vi "LoadDBCFile.vi"(10 "Signals.In":T1(array[cluster]), 11 "DbcFilePath":path caption="選擇DBC檔案") -> (1 "Signal.Out":T1(array[cluster]), 2 "Path.out":path, 3 "OK?":bool)   [LabVIEW 2024]
uses:
  LoadDBCStep.ctl
panel:
  out "Exit":bool
  in  "Signals":T1(array[cluster])
  in  "Cancel Button":bool
  in  "OK Button":bool
  in  "RemoveItem":bool
  in  "AddItem":bool
  in  "SelectedSignalName":i32(listbox) caption="顯示資料欄位"
  in  "AllSignalName":i32(listbox) caption="所有資料欄位"
  in  "LoadSignal":bool
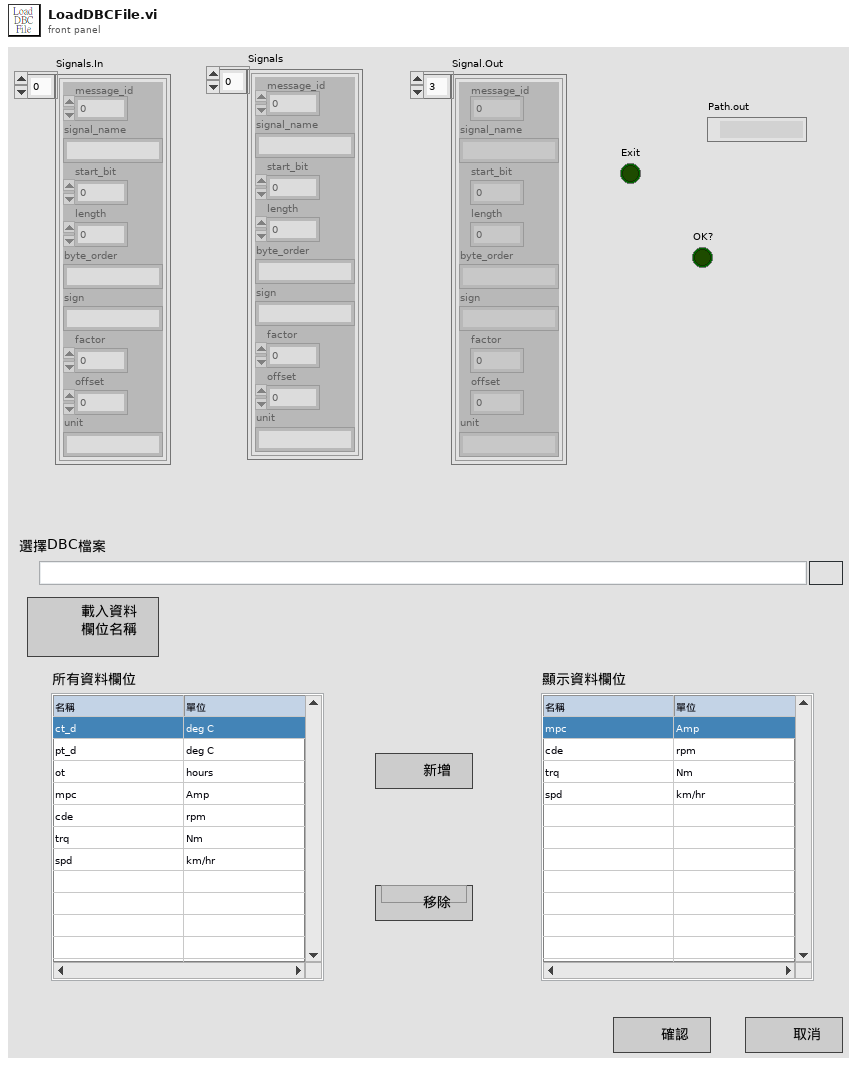
[diagram p1: front panel]
types:
  T1 = cluster{"message_id":i32, "signal_name":string, "start_bit":i32, "length":i32, "byte_order":string, "sign":string, "factor":dbl, "offset":dbl, "unit":string}[]
  T2 = typedef "LoadDBCStep.ctl" = enum16{"Idle", "Initialization", "OK Pressed", "Cancel Pressed", "LoadSignals", "AddItem", "RemoveItem", "UpdateSignalNameTable", "UpdateSelectedSignalNameTable", "End"}
  T3 = cluster{"message_id":i32, "signal_name":string, "start_bit":i32, "length":i32, "byte_order":string, "sign":string, "factor":dbl, "offset":dbl, "unit":string}
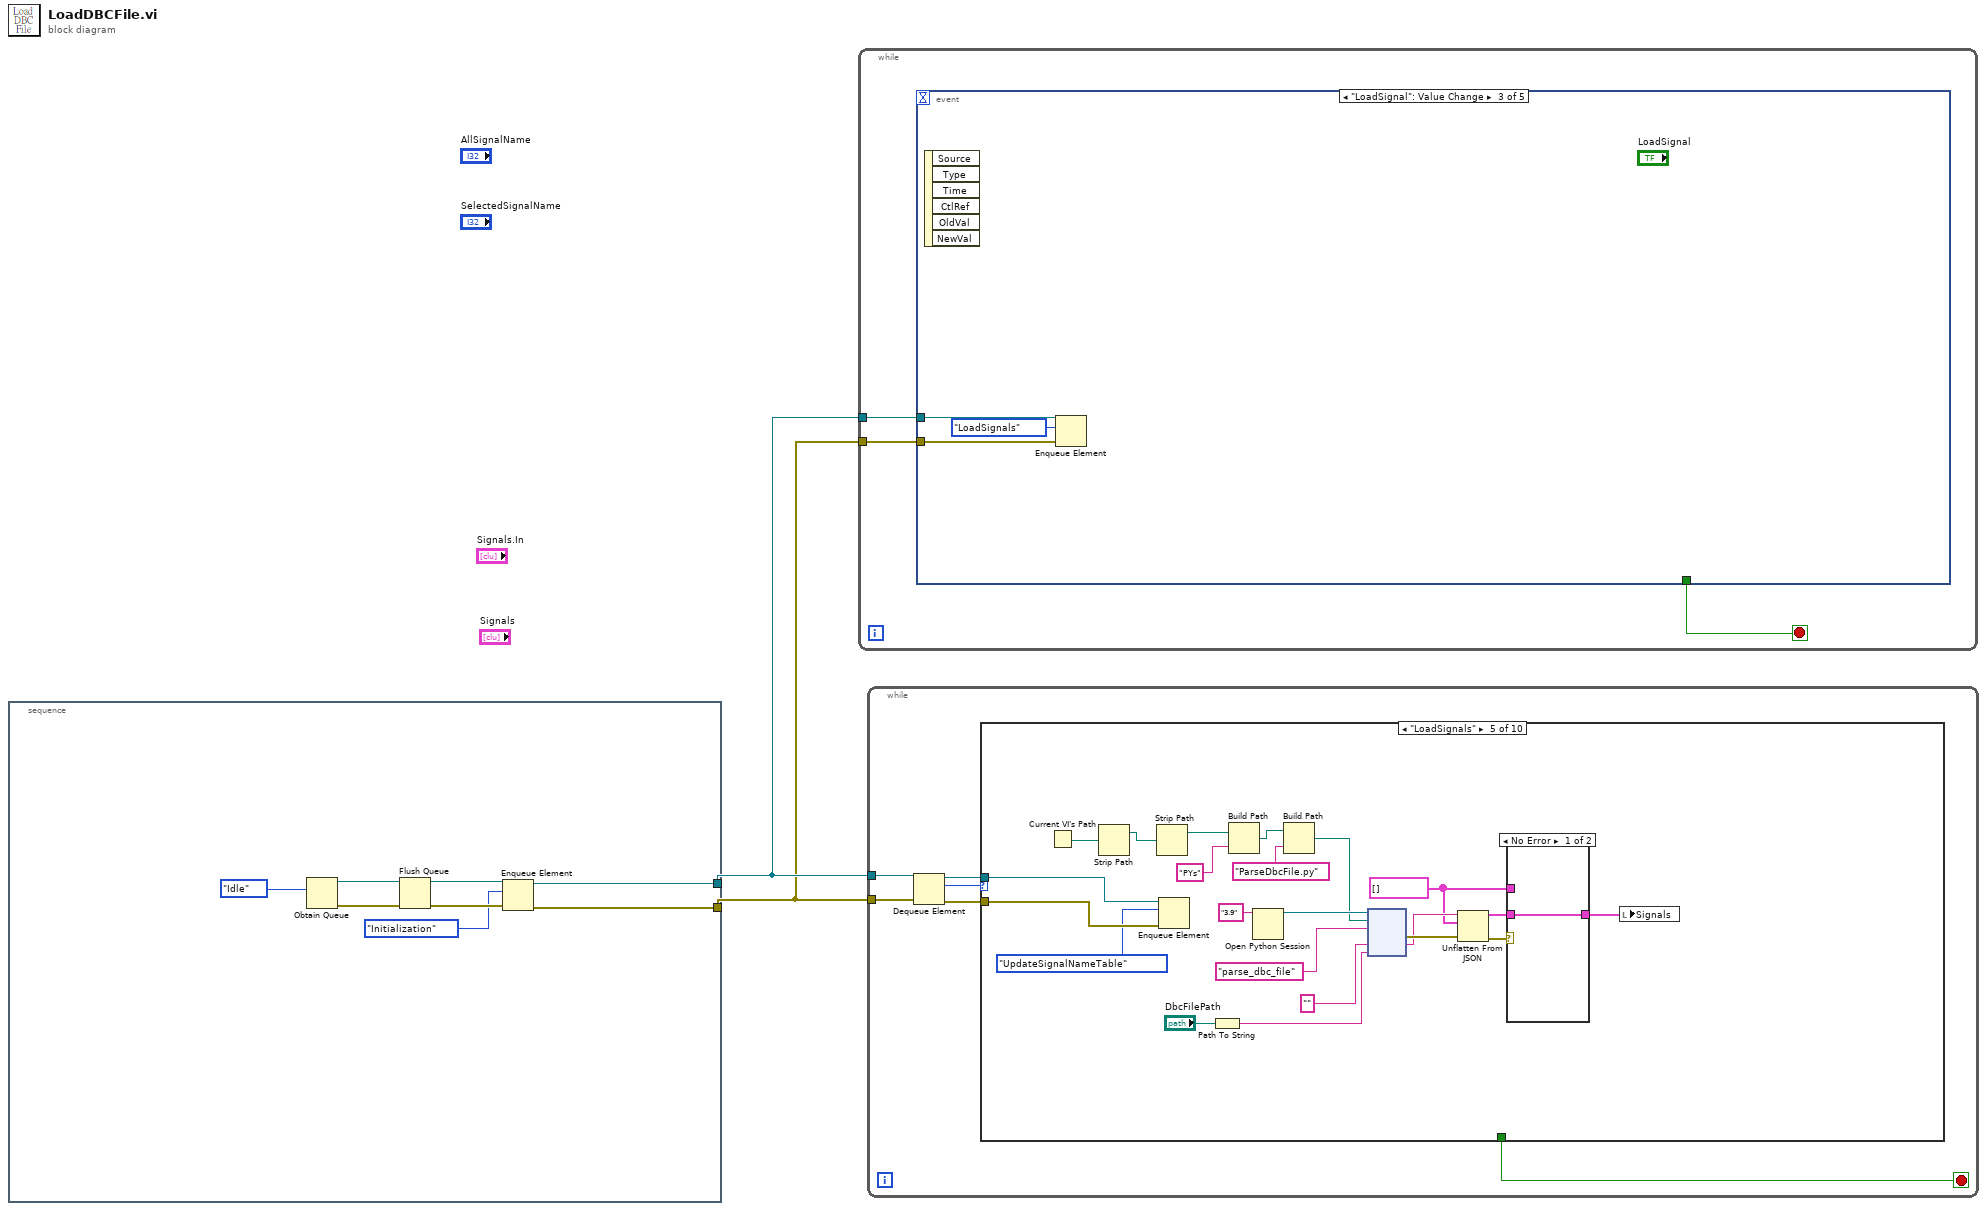
[diagram p0: block diagram]
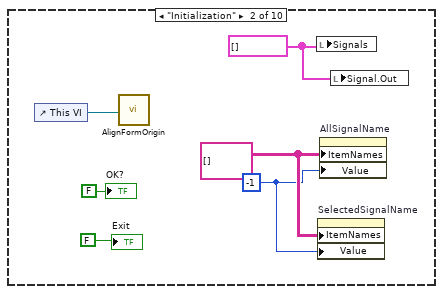
[diagram p3: hidden frame]
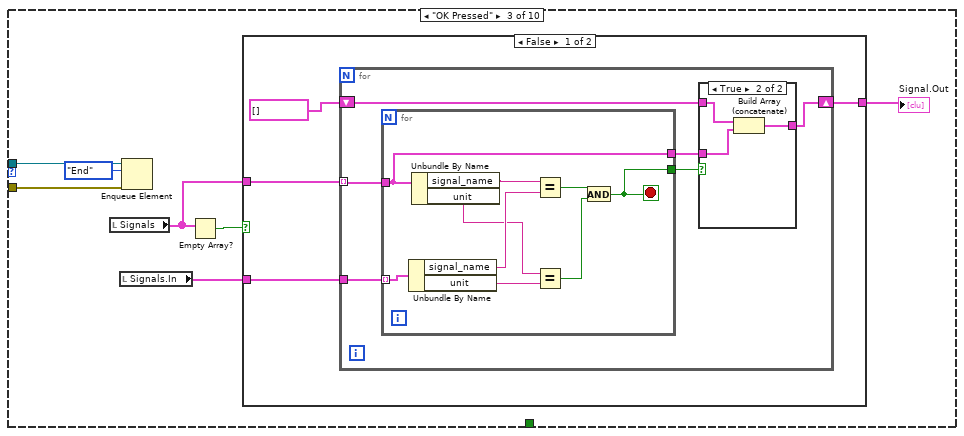
[diagram p4: hidden frame]
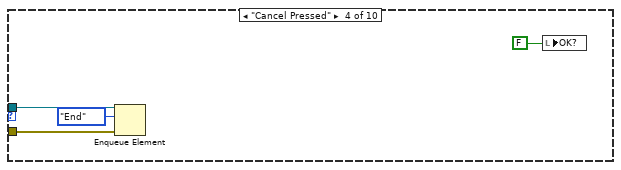
[diagram p7: hidden frame]
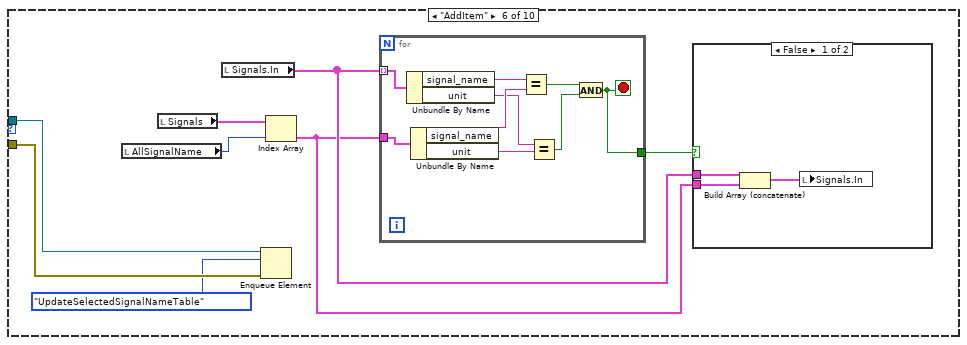
[diagram p9: hidden frame]
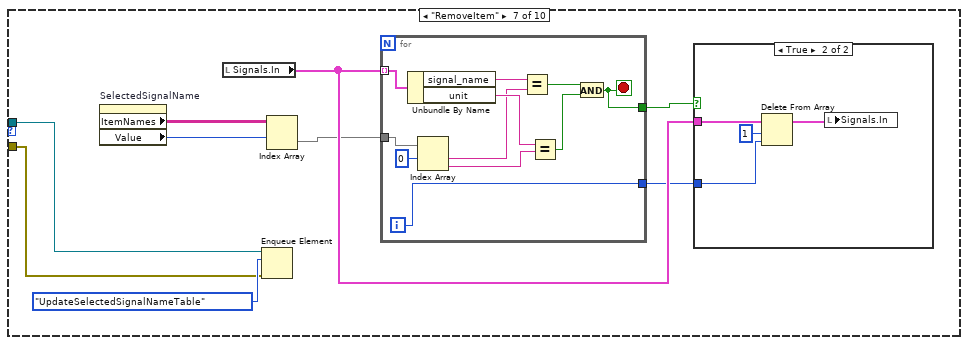
[diagram p11: hidden frame]
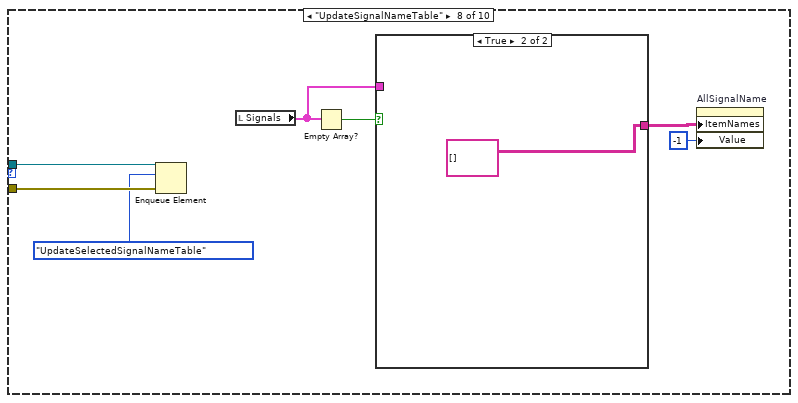
[diagram p13: hidden frame]
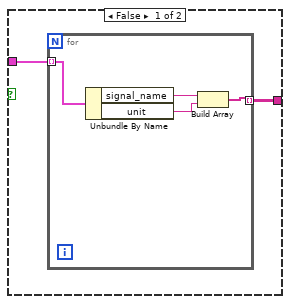
[diagram p14: hidden frame]
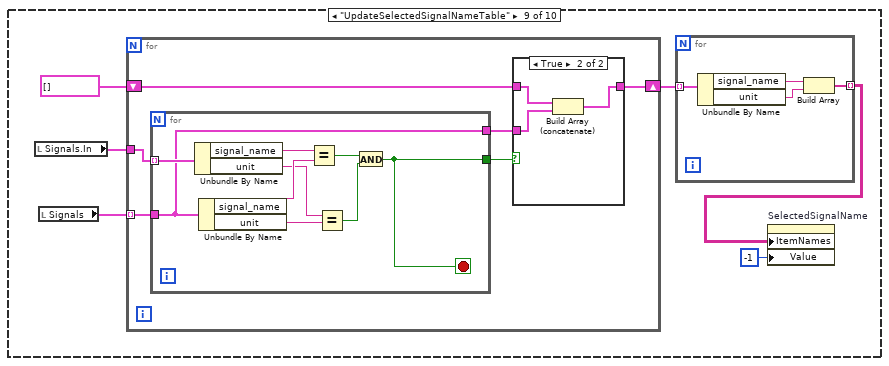
[diagram p15: hidden frame]
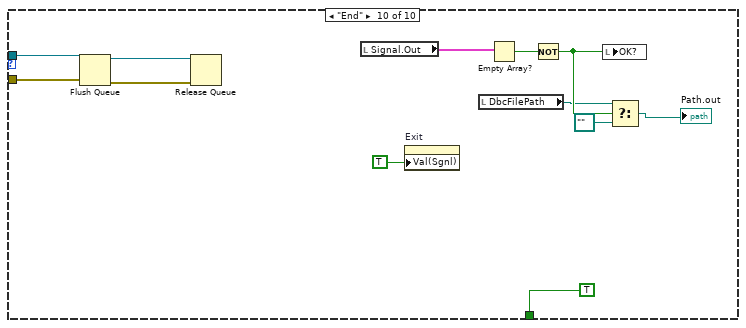
[diagram p17: hidden frame]
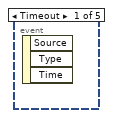
[diagram p18: hidden frame]
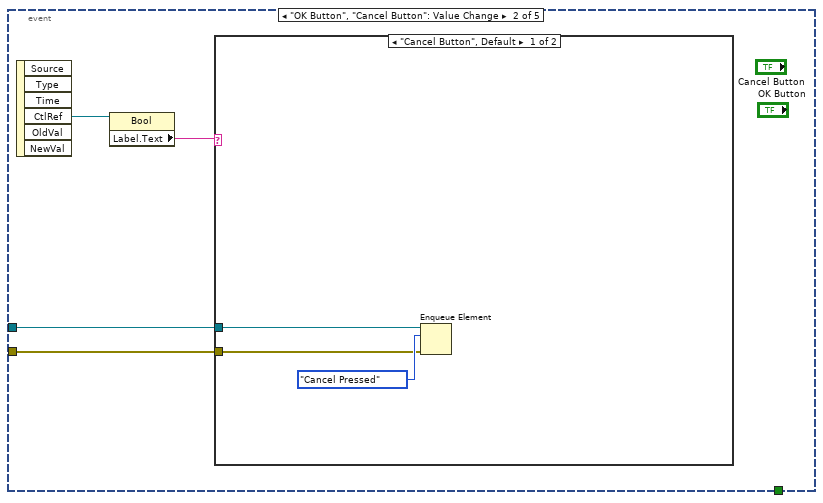
[diagram p19: hidden frame]
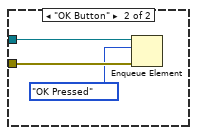
[diagram p20: hidden frame]
diagram:
  n1 = stacked-sequence {
    tunnel: [w6] -> w2
    tunnel: [w5] -> w1
    frame #0 {
      n2 = Obtain Queue(element data type=LoadDBCStep."Idle" ("Enum")) -> (queue out=w10:refnum<queue>, error out=w9:errorcluster)  [unwired: 4 in, 1 out]
      n3 = Flush Queue(queue=w10, error in (no error)=w9) -> (queue out=w8:refnum<queue>, error out=w7:errorcluster)  [unwired: 1 out]
      n4 = Enqueue Element(queue=w8, element=LoadDBCStep."Initialization", error in (no error)=w7) -> (queue out=w6:refnum<queue>, error out=w5:errorcluster)  [unwired: 1 in, 1 out]
    }
  }
  n5 = while {
    tunnel: w2 -> [w13]
    tunnel: w1 -> [w12]
    stop <- w11 stop-if-true
    n6 = event shown="[2] \"LoadSignal\": Value Change" {
      selector: _ -> [_ _ _ _ _]
      dyn-events: _ -> [_ _ _ _ _]
      timeout: _ -> [_ _ _ _ _]
      tunnel: w13 -> [_ w15 w26 w29 _]
      tunnel: w12 -> [_ w14 w25 w28 _]
      tunnel: [_ _ _ _ TRUE] -> w11
      event Timeout {
        n7 = event-data() -> ()  [unwired: 1 in, 3 out]
      }
      event "OK Button", "Cancel Button": Value Change {
        n8 = event-data() -> ("CtlRef"=w17:refnum<vi>)  [unwired: 1 in, 5 out]
        n9 = property class="Bool"(reference=w17) -> ("Label.Text"=w16:string)  [unwired: 1 in, 2 out]
        n10 = case shown="\"Cancel Button\", Default" w16 {
          tunnel: w15 -> [w19 w23]
          tunnel: w14 -> [w18 w22]
          frame "Cancel Button", Default {
            n11 = Enqueue Element(queue=w19, element=LoadDBCStep."Cancel Pressed", error in (no error)=w18) -> ()  [unwired: 1 in, 3 out]
          }
          frame "OK Button" {
            n12 = Enqueue Element(queue=w23, element=LoadDBCStep."OK Pressed", error in (no error)=w22) -> ()  [unwired: 1 in, 3 out]
          }
        }
      }
      event "LoadSignal": Value Change {
        n13 = event-data() -> ()  [unwired: 1 in, 6 out]
        n14 = Enqueue Element(queue=w26, element=LoadDBCStep."LoadSignals", error in (no error)=w25) -> ()  [unwired: 1 in, 3 out]
      }
      event "AddItem", "RemoveItem": Value Change {
        n15 = event-data() -> ("CtlRef"=w31:refnum<vi>)  [unwired: 1 in, 5 out]
        n16 = property class="Bool"(reference=w31) -> ("Label.Text"=w30:string)  [unwired: 1 in, 2 out]
        n17 = case shown="\"RemoveItemalse\", Default" w30 {
          tunnel: [LoadDBCStep."RemoveItem" ("element") LoadDBCStep."AddItem" ("element")] -> w27
          frame "RemoveItemalse", Default {
          }
          frame "AddItem" {
          }
        }
        n18 = Enqueue Element(queue=w29, element=w27, error in (no error)=w28) -> ()  [unwired: 1 in, 3 out]
      }
      event "Exit": Value Change {
        n19 = event-data() -> ()  [unwired: 1 in, 6 out]
      }
    }
  }
  n20 = while {
    tunnel: w2 -> [w40]
    tunnel: w1 -> [w39]
    stop <- w36 stop-if-true
    n21 = Dequeue Element(queue=w40, error in (no error)=w39) -> (queue out=w38:refnum<queue>, element=w35:T2, error out=w37:errorcluster)  [unwired: 1 in, 1 out]
    n22 = case shown="\"LoadSignals\"" w35 {
      tunnel: w38 -> [_ _ w49 w79 w83 w107 w129 w151 _ w203]
      tunnel: w37 -> [_ _ w48 w78 w82 w106 w130 w150 _ w202]
      tunnel: [_ _ _ _ _ _ _ _ _ TRUE] -> w36
      frame "Idle", Default {
      }
      frame "Initialization" {
        w41 = -1 ("AllSignalName")
        w42 = string[][] [] ("Item Names")
        w43 = T1 [] ("Signals")
        n23 = control-ref of="This VI"() -> (w46:refnum<vi>)
        n24 = call "AlignFormOrigin.vi"("This VI"=w46) -> ()
        n25 = local write "Signals"(w43) -> ()
        n26 = property on="SelectedSignalName" class="MCListbox (strict)"("ItemNames"=w42, "Value"=w41) -> ()  [unwired: 2 in, 2 out]
        n27 = property on="AllSignalName" class="MCListbox (strict)"("ItemNames"=w42, "Value"=w41) -> ()  [unwired: 2 in, 2 out]
        n28 = local write "Signal.Out"(w43) -> ()
        "OK?" <- FALSE ("OK?")
        "Exit" <- FALSE
      }
      frame "OK Pressed" {
        n29 = local read "Signals"() -> (w52:T1)
        n30 = local read "Signals.In"() -> (w51:T1)
        n31 = Enqueue Element(queue=w49, element=LoadDBCStep."End", error in (no error)=w48) -> ()  [unwired: 1 in, 3 out]
        n32 = Empty Array?(array=w52) -> (empty?=w53:bool)
        n33 = case shown="False" w53 {
          tunnel: w52 -> [w57 _]
          tunnel: w51 -> [w56 _]
          tunnel: [w54 _] -> w50
          frame False {
            n34 = for {
              tunnel: w57 -> [w63] mode=indexing
              tunnel: w56 -> [w62]
              shift-right: [w58] -> w54
              shift-left: T1 [] ("Signal.Out") -> [w59]
              n35 = for {
                tunnel: w63 -> [w69]
                tunnel: w62 -> [w76] mode=indexing
                tunnel: [w69] -> w60
                tunnel: [w68] -> w61
                stop <- w68 stop-if-true
                n36 = Unbundle By Name(w76) -> ("signal_name"=w74:string, "unit"=w73:string)
                n37 = Unbundle By Name(w69) -> ("signal_name"=w75:string, "unit"=w72:string)
                n38 = Equal?(x=w75, y=w74) -> (x = y?=w71:bool)
                n39 = Equal?(x=w72, y=w73) -> (x = y?=w70:bool)
                n40 = And(x=w71, y=w70) -> (x .and. y?=w68:bool)
              }
              n41 = case shown="True" w61 {
                tunnel: w60 -> [_ w66]
                tunnel: w59 -> [w64 w67]
                tunnel: [w64 w65] -> w58
                frame False {
                }
                frame True {
                  n42 = Build Array (concatenate)(w67, w66) -> (w65:T1)
                }
              }
            }
          }
          frame True {
          }
        }
        "Signal.Out" <- w50
      }
      frame "Cancel Pressed" {
        n43 = Enqueue Element(queue=w79, element=LoadDBCStep."End", error in (no error)=w78) -> ()  [unwired: 1 in, 3 out]
        n44 = local write "OK?"(FALSE) -> ()
      }
      frame "LoadSignals" {
        w84 = T1 [] ("Signals")
        n45 = Current VI's Path() -> (path=w98:path)
        n46 = Strip Path(path=w98) -> (stripped path=w97:path)  [unwired: 1 out]
        n47 = Strip Path(path=w97) -> (stripped path=w96:path)  [unwired: 1 out]
        n48 = Enqueue Element(queue=w83, element=LoadDBCStep."UpdateSignalNameTable", error in (no error)=w82) -> ()  [unwired: 1 in, 3 out]
        n49 = Path To String(path="DbcFilePath") -> (string=w90:string)
        n50 = Build Path(base path=w96, name or relative path="PYs") -> (appended path=w94:path)
        n51 = Open Python Session(python version="3.9" ("Python version")) -> (session out=w101:refnum<k35>)  [unwired: 2 in, 1 out]
        n52 = Build Path(base path=w94, name or relative path="ParseDbcFile.py") -> (appended path=w92:path)
        n53 = node(w101, w92, "parse_dbc_file" ("function name"), "", w90) -> (w89:errorcluster, w88:string)  [unwired: 2 in, 3 out]
        n54 = Unflatten From JSON(JSON string=w88, type and defaults=w84, error in (no error)=w89) -> (value=w86:T1, error out=w87:errorcluster)  [unwired: 4 in]
        n55 = case shown="No Error" w87 {
          tunnel: w86 -> [w103 _]
          tunnel: [w103 w104] -> w85
          tunnel: w84 -> [_ w104]
          frame No Error {
          }
          frame Error {
          }
        }
        n56 = local write "Signals"(w85) -> ()
      }
      frame "AddItem" {
        n57 = local read "AllSignalName"() -> (w111:i32)
        n58 = local read "Signals"() -> (w112:T1)
        n59 = local read "Signals.In"() -> (w109:T1)
        n60 = Enqueue Element(queue=w107, element=LoadDBCStep."UpdateSelectedSignalNameTable", error in (no error)=w106) -> ()  [unwired: 1 in, 3 out]
        n61 = Index Array(array=w112, index=w111) -> (element=w108:T3)
        n62 = for {
          tunnel: w109 -> [w120] mode=indexing
          tunnel: w108 -> [w119]
          tunnel: [w116] -> w110
          stop <- w116 stop-if-true
          n63 = Unbundle By Name(w120) -> ("signal_name"=w124:string, "unit"=w121:string)
          n64 = Unbundle By Name(w119) -> ("signal_name"=w123:string, "unit"=w122:string)
          n65 = Equal?(x=w124, y=w123) -> (x = y?=w118:bool)
          n66 = Equal?(x=w121, y=w122) -> (x = y?=w117:bool)
          n67 = And(x=w118, y=w117) -> (x .and. y?=w116:bool)
        }
        n68 = case shown="False" w110 {
          tunnel: w109 -> [w115 _]
          tunnel: w108 -> [w114 _]
          frame False {
            n69 = Build Array (concatenate)(w115, w114) -> (w113:T1)
            n70 = local write "Signals.In"(w113) -> ()
          }
          frame True {
          }
        }
      }
      frame "RemoveItem" {
        n71 = property on="SelectedSignalName" class="MCListbox (strict)"() -> ("ItemNames"=w128:string[][], "Value"=w127:i32)  [unwired: 2 in, 2 out]
        n72 = local read "Signals.In"() -> (w132:T1)
        n73 = Enqueue Element(queue=w129, element=LoadDBCStep."UpdateSelectedSignalNameTable", error in (no error)=w130) -> ()  [unwired: 1 in, 3 out]
        n74 = Index Array(array=w128, index (row)=w127) -> (element=w126:string[])  [unwired: 1 in]
        n75 = for {
          tunnel: w132 -> [w146] mode=indexing
          tunnel: w126 -> [w142]
          tunnel: [w143] -> w133
          tunnel: [w138] -> w125
          i -> [w138]
          stop <- w143 stop-if-true
          n76 = Unbundle By Name(w146) -> ("signal_name"=w148:string, "unit"=w147:string)
          n77 = Index Array(array=w142, index #1=0 ("index")) -> (element #1=w140:string, element #2=w139:string)  [unwired: 1 in]
          n78 = Equal?(x=w148, y=w140) -> (x = y?=w145:bool)
          n79 = Equal?(x=w147, y=w139) -> (x = y?=w144:bool)
          n80 = And(x=w145, y=w144) -> (x .and. y?=w143:bool)
        }
        n81 = case shown="True" w133 {
          tunnel: w132 -> [_ w137]
          tunnel: w125 -> [_ w135]
          frame False {
          }
          frame True {
            n82 = Delete From Array(array=w137, length=1, index=w135) -> (array with subset deleted=w134:T1)  [unwired: 1 out]
            n83 = local write "Signals.In"(w134) -> ()
          }
        }
      }
      frame "UpdateSignalNameTable" {
        n84 = Enqueue Element(queue=w151, element=LoadDBCStep."UpdateSelectedSignalNameTable", error in (no error)=w150) -> ()  [unwired: 1 in, 3 out]
        n85 = local read "Signals"() -> (w154:T1)
        n86 = Empty Array?(array=w154) -> (empty?=w155:bool)
        n87 = case shown="True" w155 {
          tunnel: w154 -> [w157 _]
          tunnel: [w156 string[][] [] ("Item Names")] -> w153
          frame False {
            n88 = for {
              tunnel: w157 -> [w161] mode=indexing
              tunnel: [w158] -> w156 mode=indexing
              n89 = Unbundle By Name(w161) -> ("signal_name"=w160:string, "unit"=w159:string)
              n90 = Build Array(w160, w159) -> (w158:string[])
            }
          }
          frame True {
          }
        }
        n91 = property on="AllSignalName" class="MCListbox (strict)"("ItemNames"=w153, "Value"=-1 ("AllSignalName")) -> ()  [unwired: 2 in, 2 out]
      }
      frame "UpdateSelectedSignalNameTable" {
        n92 = local read "Signals.In"() -> (w168:T1)
        n93 = local read "Signals"() -> (w167:T1)
        n94 = for {
          tunnel: w168 -> [w177]
          tunnel: w167 -> [w178] mode=indexing
          shift-right: [w174] -> w165
          shift-left: T1 [] ("Signal.Out") -> [w175]
          n95 = for {
            tunnel: w178 -> [w183]
            tunnel: w177 -> [w191] mode=indexing
            tunnel: [w184] -> w176
            tunnel: [w183] -> w173
            stop <- w184 stop-if-true
            n96 = Unbundle By Name(w191) -> ("signal_name"=w190:string, "unit"=w187:string)
            n97 = Unbundle By Name(w183) -> ("signal_name"=w189:string, "unit"=w188:string)
            n98 = Equal?(x=w190, y=w189) -> (x = y?=w186:bool)
            n99 = Equal?(x=w187, y=w188) -> (x = y?=w185:bool)
            n100 = And(x=w186, y=w185) -> (x .and. y?=w184:bool)
          }
          n101 = case shown="True" w176 {
            tunnel: w175 -> [w179 w182]
            tunnel: [w179 w181] -> w174
            tunnel: w173 -> [_ w180]
            frame False {
            }
            frame True {
              n102 = Build Array (concatenate)(w182, w180) -> (w181:T1)
            }
          }
        }
        n103 = for {
          tunnel: w165 -> [w172] mode=indexing
          tunnel: [w169] -> w164 mode=indexing
          n104 = Unbundle By Name(w172) -> ("signal_name"=w171:string, "unit"=w170:string)
          n105 = Build Array(w171, w170) -> (w169:string[])
        }
        n106 = property on="SelectedSignalName" class="MCListbox (strict)"("ItemNames"=w164, "Value"=-1 ("SelectedSignalName")) -> ()  [unwired: 2 in, 2 out]
      }
      frame "End" {
        n107 = Flush Queue(queue=w203, error in (no error)=w202) -> (queue out=w201:refnum<queue>, error out=w200:errorcluster)  [unwired: 1 out]
        n108 = Release Queue(queue=w201, error in (no error)=w200) -> ()  [unwired: 1 in, 3 out]
        n109 = local read "Signal.Out"() -> (w197:T1)
        n110 = property on="Exit" class="Bool (strict)"("Val(Sgnl)"=TRUE) -> ()  [unwired: 2 in, 2 out]
        n111 = local read "DbcFilePath"() -> (w194:path)
        n112 = Empty Array?(array=w197) -> (empty?=w196:bool)
        n113 = Not(x=w196) -> (.not. x?=w195:bool)
        n114 = local write "OK?"(w195) -> ()
        n115 = Select(t=w194, s=w195, f=path "") -> (s? t:f=→"Path.out":path)
      }
    }
  }
